vi "SensorOperation.vi"(4 "SystemLink":T1={"APIKey"="", "Tag"="", "Type"="STRING"}, 6 "WiFi":cluster{"SSID":string, "Key":string}, 8 "ROI":string="r=[%d,%d,%d,%d]", 9 "Lab":string="[(0,100,-127,128,-127,128)]", 10 "Destination":T2(ring), 11 "View":T3(ring)) -> (3 "startCode":string)   [LabVIEW 2016]
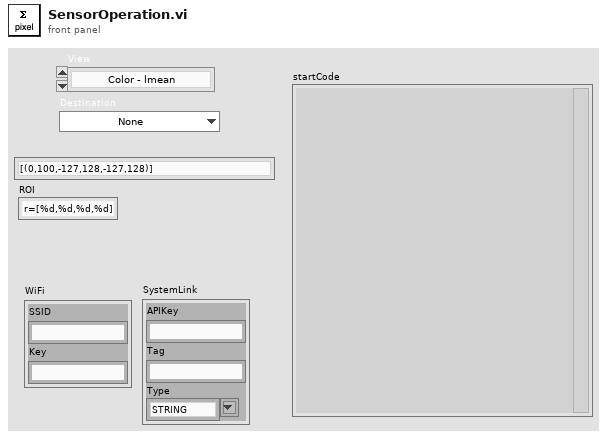
[diagram p1: front panel]
types:
  T1 = cluster{"APIKey":string, "Tag":string, "Type":string}
  T2 = enum16{"None", "UART (Tx-4, Rx-5)", "SPI (MOSI - 0, MISO-1, SCK-2)", "I2C (SCL-4,SDA-5)", "WiFi"}
  T3 = enum16{"Color - lmean", "Color - lmode", "Greyscale - mean", "Greyscale - mode", "Track Blobs", "Track Faces", "QRCode"}
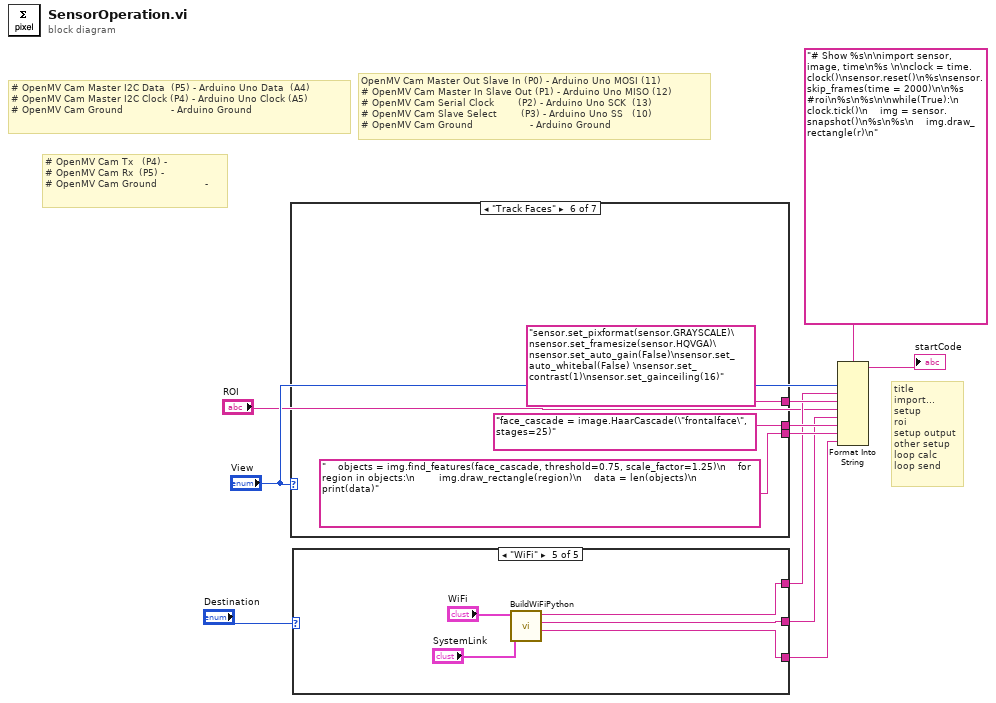
[diagram p0: block diagram]
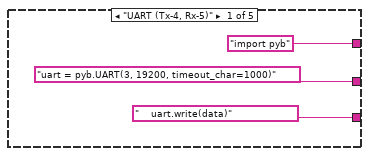
[diagram p2: hidden frame]
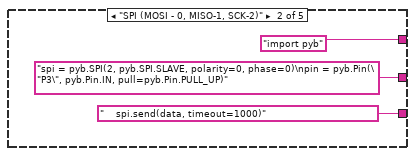
[diagram p3: hidden frame]
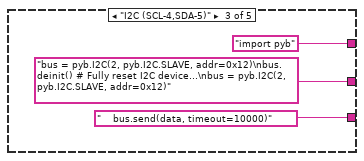
[diagram p4: hidden frame]
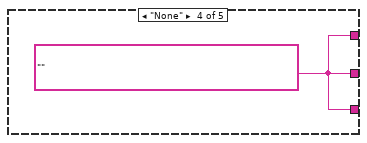
[diagram p5: hidden frame]
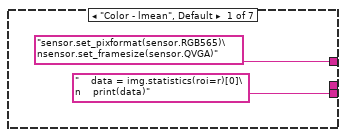
[diagram p6: hidden frame]
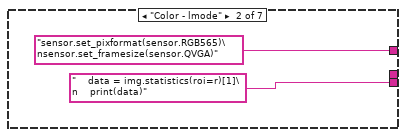
[diagram p7: hidden frame]
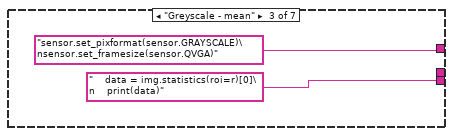
[diagram p8: hidden frame]
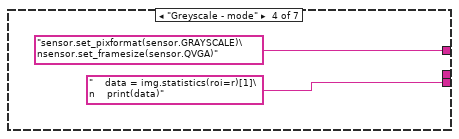
[diagram p9: hidden frame]
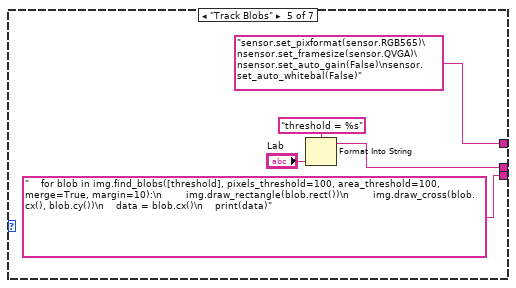
[diagram p10: hidden frame]
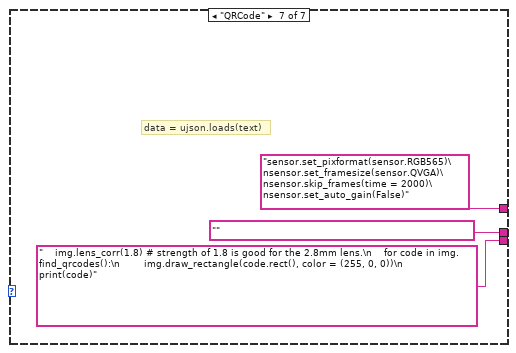
[diagram p11: hidden frame]
diagram:
  # "title\nimport...\nsetup\nroi\nsetup output\nother setup\nloop calc\nloop send"
  # "# OpenMV Cam Tx   (P4) -\n# OpenMV Cam Rx  (P5) - \n# OpenMV Cam Ground                -"
  # "# OpenMV Cam Master I2C Data  (P5) - Arduino Uno Data  (A4)\n# OpenMV Cam Master I2C Clock (P4) - Arduino Uno Clock (A5)\n# OpenMV Cam Ground                - Arduino Ground"
  # "OpenMV Cam Master Out Slave In (P0) - Arduino Uno MOSI (11)\n# OpenMV Cam Master In Slave Out (P1) - Arduino Uno MISO (12)\n# OpenMV Cam Serial Clock        (P2) - Arduino Uno SCK  (13)\n# OpenMV Cam Slave Select        (P3) - Arduino Uno SS   (10)\n# OpenMV Cam Ground                   - Arduino Ground"
  n1 = case shown="\"Track Faces\"" "View" {
    tunnel: ["    data = img.statistics(roi=r)[0]\n    print(data)" "    data = img.statistics(roi=r)[1]\n    print(data)" "    data = img.statistics(roi=r)[0]\n    print(data)" "    data = img.statistics(roi=r)[1]\n    print(data)" "    for blob in img.find_blobs([threshold], pixels_threshold=100, area_threshold=100, merge=True, margin=10):\n        img.draw_rectangle(blob.rect())\n        img.draw_cross(blob.cx(), blob.cy())\n    data = blob.cx()\n    print(data)" "    objects = img.find_features(face_cascade, threshold=0.75, scale_factor=1.25)\n    for region in objects:\n        img.draw_rectangle(region)\n    data = len(objects)\n    print(data)" "    img.lens_corr(1.8) # strength of 1.8 is good for the 2.8mm lens.\n    for code in img.find_qrcodes():\n        img.draw_rectangle(code.rect(), color = (255, 0, 0))\n        print(code)"] -> w7
    tunnel: ["sensor.set_pixformat(sensor.RGB565)\nsensor.set_framesize(sensor.QVGA)" ("startCode") "sensor.set_pixformat(sensor.RGB565)\nsensor.set_framesize(sensor.QVGA)" ("startCode") "sensor.set_pixformat(sensor.GRAYSCALE)\nsensor.set_framesize(sensor.QVGA)" ("startCode") "sensor.set_pixformat(sensor.GRAYSCALE)\nsensor.set_framesize(sensor.QVGA)" ("startCode") "sensor.set_pixformat(sensor.RGB565)\nsensor.set_framesize(sensor.QVGA)\nsensor.set_auto_gain(False)\nsensor.set_auto_whitebal(False)" ("startCode") "sensor.set_pixformat(sensor.GRAYSCALE)\nsensor.set_framesize(sensor.HQVGA)\nsensor.set_auto_gain(False)\nsensor.set_auto_whitebal(False) \nsensor.set_contrast(1)\nsensor.set_gainceiling(16)" ("startCode") "sensor.set_pixformat(sensor.RGB565)\nsensor.set_framesize(sensor.QVGA)\nsensor.skip_frames(time = 2000)\nsensor.set_auto_gain(False)" ("startCode")] -> w9
    tunnel: [_ _ _ _ w22 "face_cascade = image.HaarCascade(\"frontalface\", stages=25)" ""] -> w8
    frame "Color - lmean", Default {
    }
    frame "Color - lmode" {
    }
    frame "Greyscale - mean" {
    }
    frame "Greyscale - mode" {
    }
    frame "Track Blobs" {
      n2 = Format Into String(format string="threshold = %s", "Lab") -> (resulting string=w22:string)  [unwired: 2 in, 1 out]
    }
    frame "Track Faces" {
    }
    frame "QRCode" {
      # "data = ujson.loads(text)"
    }
  }
  n3 = case shown="\"WiFi\"" "Destination" {
    tunnel: ["uart = pyb.UART(3, 19200, timeout_char=1000)" "spi = pyb.SPI(2, pyb.SPI.SLAVE, polarity=0, phase=0)\npin = pyb.Pin(\"P3\", pyb.Pin.IN, pull=pyb.Pin.PULL_UP)" "bus = pyb.I2C(2, pyb.I2C.SLAVE, addr=0x12)\nbus.deinit() # Fully reset I2C device...\nbus = pyb.I2C(2, pyb.I2C.SLAVE, addr=0x12)" w40 w43] -> w5
    tunnel: ["    uart.write(data)" "    spi.send(data, timeout=1000)" "    bus.send(data, timeout=10000)" w40 w45] -> w4
    tunnel: ["import pyb" "import pyb" "import pyb" w40 w42] -> w2
    frame "UART (Tx-4, Rx-5)" {
    }
    frame "SPI (MOSI - 0, MISO-1, SCK-2)" {
    }
    frame "I2C (SCL-4,SDA-5)" {
    }
    frame "None" {
      w40 = ""
    }
    frame "WiFi" {
      n4 = call "BuildWiFiPython.vi"("SystemLink"="SystemLink", "WiFi"="WiFi") -> ("Repeated call"=w45:string, "Setup"=w43:string, "Headers"=w42:string)  [unwired: 7 in]
    }
  }
  n5 = Format Into String(format string="# Show %s\n\nimport sensor, image, time\n%s \n\nclock = time.clock()\nsensor.reset()\n%s\nsensor.skip_frames(time = 2000)\n\n%s  #roi\n%s\n%s\n\nwhile(True):\n    clock.tick()\n    img = sensor.snapshot()\n%s\n%s\n    img.draw_rectangle(r)\n" ("startCode"), "View", w2, w9, "ROI", w5, w8, w7, w4) -> (resulting string=→"startCode":string)  [unwired: 2 in, 1 out]
